vi "String to Boolean_csm.vi"(1 "Default (F)":bool, 3 "String":string) -> (0 "Boolean":bool)   [LabVIEW 2017, in "API String Arguments Support.lvlib"]
doc: "Converts a string to a boolean value. Supports multiple representations for TRUE/FALSE. Custom TRUE/FALSE strings can be added via the API String - Add Boolean Strings VI.\n\n\n> [!NOTE] <b>Default Strings for TRUE Value</b>\n>\n> Supports `1`, `Active`, `Enable`, `Non-null`, `On`, `T`, `True`, `valid`, `yes`.\n>\n> Case insensitive.\n\n\n> [!NOTE] <b>Default Strings for FALSE Value</b>\n>\n> Supports `0`, `Disable`, `F`, `False`, `Inactive`, `Invalid`, `No`, `Off`, `Void`, `null`.\n>\n> Case insensitive.\n\n\n-- <b>Controls</b> --\n- <b>String</b>: Input string.\n- <b>Default (F)</b>: Default value if conversion fails.\n\n-- <b>Indicators</b> --\n- <b>Boolean</b>: Converted boolean value."
uses:
  API String Arguments Support.lvlib
  <userlib>/_NEVSTOP/Communicable State Machine(CSM)/_Shared/CSM Shared.lvlib
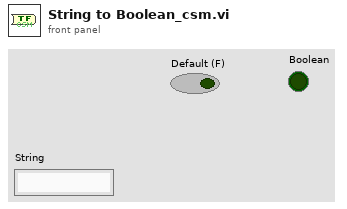
[diagram p1: front panel]
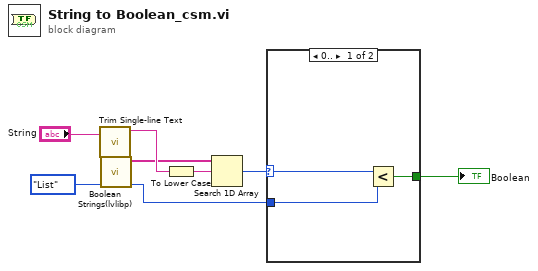
[diagram p0: block diagram]
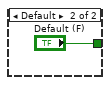
[diagram p2: hidden frame]
diagram:
  n1 = call <userlib>:"Trim Single-line Text.vi"("single-line text"="String") -> ("trimed text"=w6:string)  [unwired: 2 in]
  n2 = call "Boolean Strings(lvlibp).vi"("Enum"=enum16{"List", "Add", "Remove"}."List") -> ("Numeric"=w3:i32, "Array"=w4:string[])  [unwired: 7 in, 2 out]
  n3 = To Lower Case(string=w6) -> (all lower case string=w1:string)
  n4 = Search 1D Array(1D array=w4, element=w1) -> (index of element=w5:i32)  [unwired: 1 in]
  n5 = case shown="0.." w5 {
    selector: w5 -> [w11 _]
    tunnel: [w9 "Default (F)"] -> w7
    tunnel: w3 -> [w10 _]
    frame 0.. {
      n6 = Less?(x=w11, y=w10) -> (x < y?=w9:bool)
    }
    frame Default {
    }
  }
  "Boolean" <- w7
